vi "IDD Test_no config.vi"(6 "script name":string="IDD", 8 "error in (no error)":errorcluster, 9 "Publishable IDs":string[](array[string])=["IDD_LowPower", "IDD_DVC_Cmin", "IDD_DVC_Cmax"], 10 "Pins":string[](array[string])=["VDD"], 11 "Semiconductor Module Context":T1) -> (0 "error out":errorcluster)   [LabVIEW 2013]
uses:
  <vilib>/NI_TestStand_SemiconductorModule/NI_TestStand_Semiconductor_Module.lvlibp/PinMap/General/SemiconductorModuleContext.ctl
  <instrlib>/niHSDIO/niHSDIO.llb/niHSDIO_ctl Trigger Script - trigID Values (Ring).ctl
  <vilib>/NI_TestStand_SemiconductorModule/NI_TestStand_Semiconductor_Module.lvlibp/PinMap/DC Power/PinsToNIDCPowerSessions.vi
  <vilib>/NI_TestStand_SemiconductorModule/NI_TestStand_Semiconductor_Module.lvlibp/PinMap/General/Publish/PublishDataDouble2D.vi
  <vilib>/NI_TestStand_SemiconductorModule/NI_TestStand_Semiconductor_Module.lvlibp
panel:
  out "current measurements":dbl[][](array[numeric])
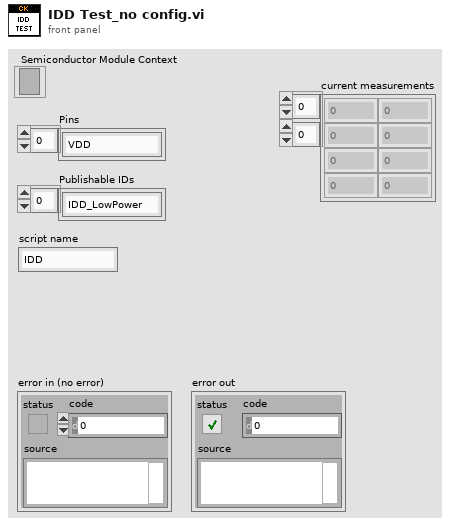
[diagram p1: front panel]
types:
  T1 = typedef "NI_TestStand_Semiconductor_Module.lvlibp/SemiconductorModuleContext.ctl" = refnum<k7>
  T2 = typedef "niHSDIO_ctl Trigger Script - trigID Values (Ring).ctl" = string
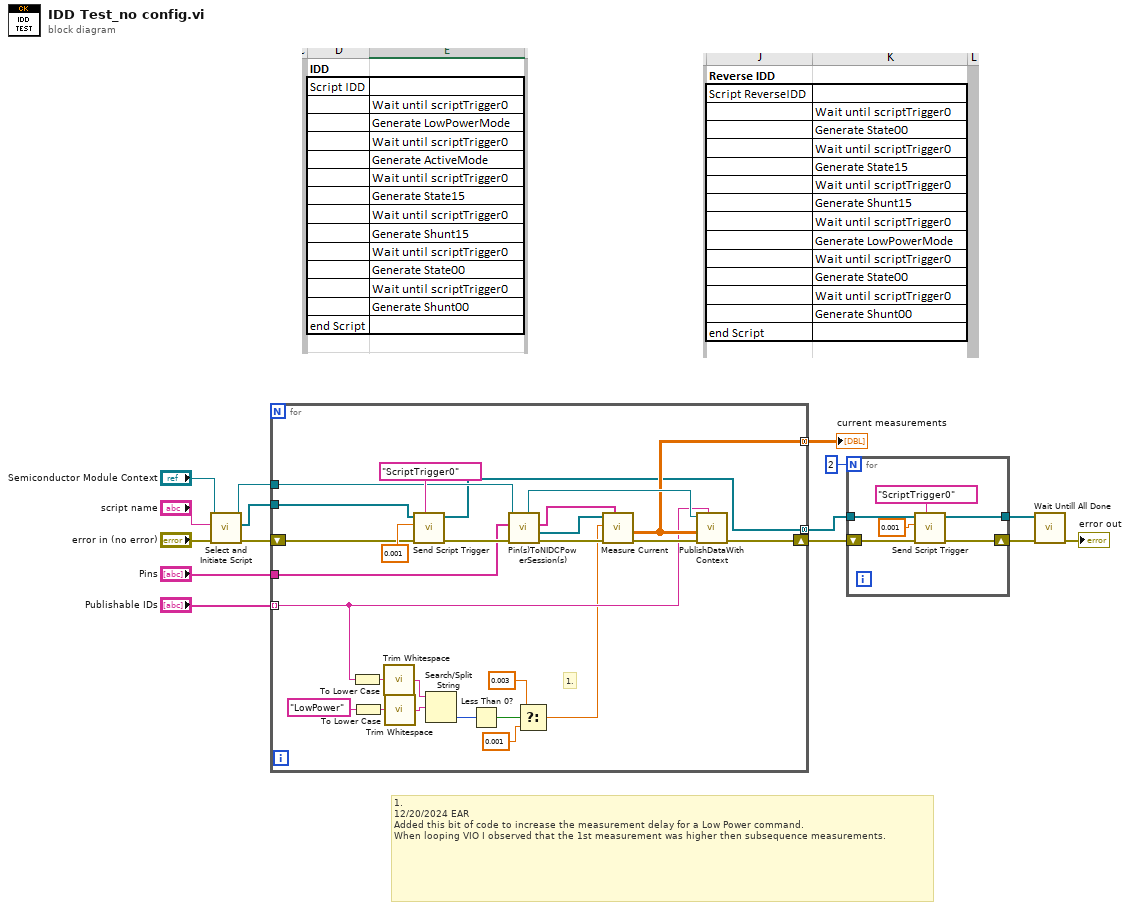
[diagram p0: block diagram]
diagram:
  # "1.\n12/20/2024 EAR\nAdded this bit of code to increase the measurement delay for a Low Power command. \nWhen looping VIO I observed that the 1st measurement was higher then subsequence measurements."
  n1 = call "Select and Initiate Script.vi"("error in (no error)"="error in (no error)", "script name"="script name", "Semiconductor Module Context"="Semiconductor Module Context") -> ("error out"=w1:errorcluster, "HSDIO GEN Sessions Out"=w10:refnum<k15>[], "Semiconductor Module Context Out"=w3:T1)  [unwired: 6 in]
  n2 = for {
    tunnel: "Pins" -> [w28]
    tunnel: w3 -> [w33]
    tunnel: w10 -> [w27]
    tunnel: "Publishable IDs" -> [w22] mode=indexing
    shift-right: [w36] -> w8
    shift-left: w1 -> [w29]
    tunnel: [w31] -> w11 mode=concatenating
    tunnel: [w30] -> w6 mode=concatenating
    # "1."
    n3 = To Lower Case(string=w22) -> (all lower case string=w26:string)
    n4 = To Lower Case(string="LowPower") -> (all lower case string=w25:string)
    n5 = call <vilib>:"Trim Whitespace.vi"("string"=w26) -> ("trimmed string"=w23:string)  [unwired: 1 in]
    n6 = call <vilib>:"Trim Whitespace.vi"("string"=w25) -> ("trimmed string"=w24:string)  [unwired: 1 in]
    n7 = call "Send Script Trigger.vi"("trigger id (script trigger 0)"=T2 "ScriptTrigger0", "error in (no error)"=w29, "Delay Time (s)"=0.001, "HSDIO Sessions In"=w27) -> ("error out"=w34:errorcluster, "HSDIO Sessions Out"=w30:refnum<k15>[])  [unwired: 6 in]
    n8 = Search/Split String(string=w23, search string/char (-)=w24) -> (offset of match=w20:i32)  [unwired: 1 in, 2 out]
    n9 = Less Than 0?(x=w20) -> (x < 0?=w19:bool)
    n10 = call-poly <vilib>:"Pin(s)ToNIDCPowerSession(s).vi"("error in (no error)"=w34, "Pins"=w28, "Semiconductor Module Context"=w33) -> ("error out"=w37:errorcluster, "Instrument Sessions"=w41:refnum<k15>[], "Channel Lists"=w39:string[], "Pin Query Context"=w38:refnum<class "MultiplePinMultipleSessionQueryContext.lvclass">)  [unwired: 4 in, 1 out]
    n11 = Select(t=0.003 ("Delay Time (s)"), s=w19, f=0.001 ("Delay Time (s)")) -> (s? t:f=w16:dbl)
    n12 = call "Measure Current.vi"("Channel Lists"=w39, "error in (no error)"=w37, "Delay Time (s)"=w16, "DCPower Sessions In"=w41) -> ("error out"=w40:errorcluster, "current measurements"=w31:dbl[][])  [unwired: 5 in, 1 out]
    n13 = call-poly <vilib>:"PublishDataWithContext.vi"("Published Data Id"=w22, "error in (no error)"=w40, "Data In"=w31, "Pin Query Context"=w38) -> ("error out"=w36:errorcluster)  [unwired: 6 in, 1 out]
  }
  "current measurements" <- w11
  n14 = for {
    N: 2 -> [_]
    tunnel: w6 -> [w45]
    tunnel: [w42] -> w5
    shift-right: [w46] -> w7
    shift-left: w8 -> [w47]
    n15 = call "Send Script Trigger.vi"("trigger id (script trigger 0)"=T2 "ScriptTrigger0", "error in (no error)"=w47, "Delay Time (s)"=0.001, "HSDIO Sessions In"=w45) -> ("error out"=w46:errorcluster, "HSDIO Sessions Out"=w42:refnum<k15>[])  [unwired: 6 in]
  }
  n16 = call "Wait Untill All Done.vi"("error in (no error)"=w7, "HSDIO Sessions In"=w5) -> ("error out"=→"error out":errorcluster)  [unwired: 8 in, 1 out]
